vi "cDAQ DDS To Idle.vi"(8 "error in":errorcluster, 11 "cDAQ dds":T1={"device"="", "channels"=[], "mclk source"="", "mclk [Hz]"=0.0, "fs [Hz]"=0.0, "block [s]"=0.0, "buf [s]"=0.0, "task"="", "cmd queue"=refnum, "proc ref"=refnum, "smpl clock out"="/cDAQ3/PFI0", "export smpl clock"=FALSE, "DC ofs [V]"=[], "timebase source"="", "timebase mode"=enum."Local"} {"channels" min=0 step=1}) -> (0 "error out":errorcluster, 3 "cDAQ dds out":T1={"device"="", "channels"=[], "mclk source"="", "mclk [Hz]"=0.0, "fs [Hz]"=0.0, "block [s]"=0.0, "buf [s]"=0.0, "task"="", "cmd queue"=refnum, "proc ref"=refnum, "smpl clock out"="/cDAQ3/PFI0", "export smpl clock"=FALSE, "DC ofs [V]"=[], "timebase source"="", "timebase mode"=enum."Local"} {"channels" min=0 step=1})   [LabVIEW 2020]
uses:
  cDAQ DDS Session.ctl
  cDAQ DDS Setup.ctl
  cDAQ DDS Timebase Mode.ctl
  <vilib>/DAQmx/write.llb/DAQmx Write (Analog 2D DBL NChan NSamp).vi
  <vilib>/DAQmx/configure/timing.llb/DAQmx Timing (Sample Clock).vi
  <vilib>/DAQmx/miscellaneous.llb/DAQmx Fill In Error Info.vi
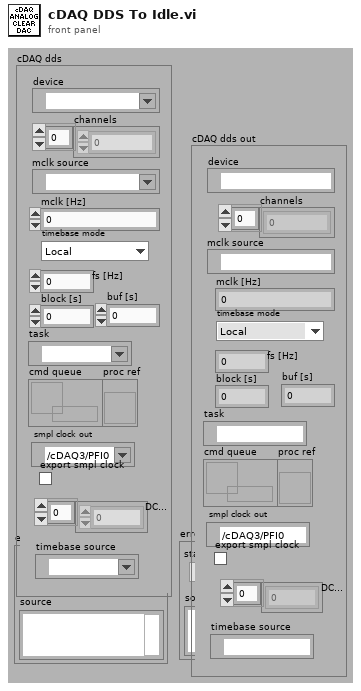
[diagram p1: front panel]
types:
  T1 = typedef "cDAQ DDS Session.ctl" = cluster{"device":tag, "channels":i32[], "mclk source":tag, "mclk [Hz]":dbl, "fs [Hz]":dbl, "block [s]":dbl, "buf [s]":dbl, "task":refnum<k21>, "cmd queue":refnum<queue>, "proc ref":refnum<vi>, "smpl clock out":tag, "export smpl clock":bool, "DC ofs [V]":dbl[], "timebase source":tag, "timebase mode":T2}
  T2 = typedef "cDAQ DDS Timebase Mode.ctl" = enum16{"Local", "Take from ADC (e.g. NI 9238)", "Other source"}
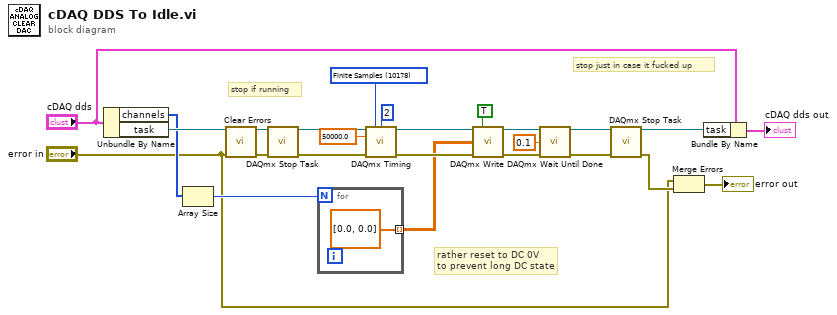
[diagram p0: block diagram]
diagram:
  w21 = 10178 items=["Finite Samples"=10178, "Continuous Samples"=10123, "Hardware Timed Single Point"=12522] ("sample mode")
  # "stop just in case it fucked up"
  # "rather reset to DC 0V\nto prevent long DC state"
  # "stop if running"
  n1 = Unbundle By Name("cDAQ dds") -> ("channels"=w8:i32[], "task"=w10:refnum<k21>)
  n2 = Array Size(array=w8) -> (size(s)=w7:i32)
  n3 = call <vilib>:"Clear Errors.vi"("error in (no error)"="error in") -> ("error out"=w9:errorcluster)  [unwired: 5 in, 1 out]
  n4 = call <vilib>:"DAQmx Stop Task.vi"("task/channels in"=w10, "error in"=w9) -> ("task out"=w13:refnum<k21>, "error out"=w12:errorcluster)  [unwired: 12 in]
  n5 = for {
    N: w7 -> [_]
    tunnel: [dbl[] [0.0, 0.0]] -> w11 mode=indexing
  }
  n6 = call-poly <vilib>:"DAQmx Timing.vi"("task/channels in"=w13, "sample mode"=w21, "samples per channel"=2, "rate"=50000.0, "error in"=w12) -> ("task out"=w24:refnum<k21>, "error out"=w20:errorcluster)  [unwired: 9 in]
  n7 = call-poly <vilib>:"DAQmx Write.vi"("task/channels in"=w24, "auto start"=TRUE, "data"=w11, "error in"=w20) -> ("task out"=w18:refnum<k21>, "error out"=w17:errorcluster)  [unwired: 9 in, 1 out]
  n8 = call <vilib>:"DAQmx Wait Until Done.vi"("task/channels in"=w18, "timeout (sec)"=0.1, "error in"=w17) -> ("task out"=w14:refnum<k21>, "error out"=w15:errorcluster)  [unwired: 11 in]
  n9 = call <vilib>:"DAQmx Stop Task.vi"("task/channels in"=w14, "error in"=w15) -> ("task out"=w2:refnum<k21>, "error out"=w6:errorcluster)  [unwired: 12 in]
  n10 = Merge Errors("error in", w6) -> (→"error out":errorcluster)
  n11 = Bundle By Name(cluster="cDAQ dds", "task"=w2) -> (→"cDAQ dds out":T1)
